vi "SerialWriteLines.vi"(8 "error in (no error)":errorcluster, 9 "REPL":string, 10 "Send":string, 11 "VISA Refnum in":refnum<visa-resource-name>) -> (0 "error out":errorcluster, 1 "Rest":string, 3 "VISA Refnum out":refnum<visa-resource-name>)   [LabVIEW 2020]
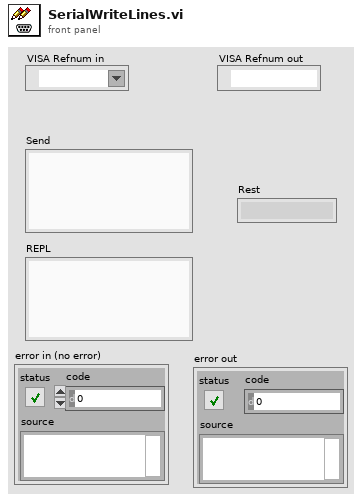
[diagram p1: front panel]
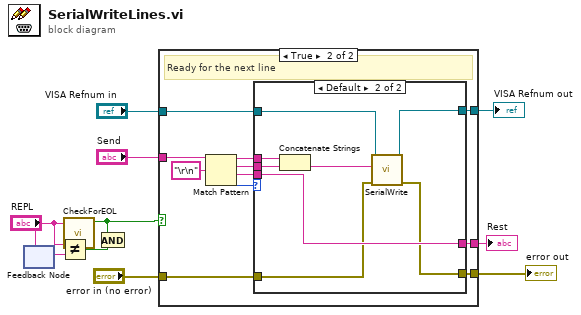
[diagram p0: block diagram]
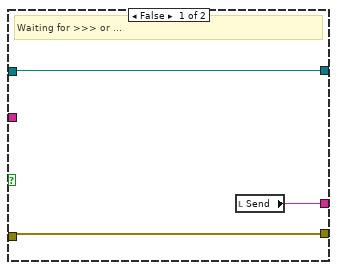
[diagram p2: hidden frame]
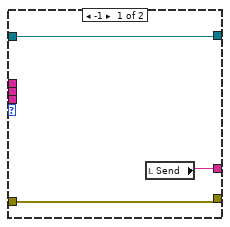
[diagram p3: hidden frame]
diagram:
  n1 = feedback-in #1("REPL") -> ()
  n2 = feedback #1() -> (w4:string)  [unwired: 1 in]
  n3 = Not Equal?(x="REPL", y=w4) -> (x != y?=w2:bool)
  n4 = call "CheckForEOL.vi"("REPL"="REPL") -> ("Complete?"=w1:bool)  [unwired: 10 in]
  n5 = And(x=w1, y=w2) -> ()  [unwired: 1 out]
  n6 = case shown="True" w1 {
    tunnel: "Send" -> [_ w23]
    tunnel: [w13 w19] -> w9
    tunnel: "VISA Refnum in" -> [w11 w17]
    tunnel: "error in (no error)" -> [w12 w16]
    tunnel: [w12 w15] -> w6
    tunnel: [w11 w14] -> w5
    frame False {
      # "Waiting for >>> or ..."
      n7 = local read "Send"() -> (w13:string)
    }
    frame True {
      # "Ready for the next line"
      n8 = Match Pattern(string=w23, regular expression="\r\n") -> (before substring=w24:string, match substring=w22:string, after substring=w18:string, offset past match=w20:i32)  [unwired: 1 in]
      n9 = case shown="Default" w20 {
        tunnel: w24 -> [_ w35]
        tunnel: w22 -> [_ w34]
        tunnel: w17 -> [w25 w32]
        tunnel: [w27 w33] -> w19
        tunnel: w18 -> [_ w33]
        tunnel: w16 -> [w26 w29]
        tunnel: [w26 w28] -> w15
        tunnel: [w25 w31] -> w14
        frame -1 {
          n10 = local read "Send"() -> (w27:string)
        }
        frame Default {
          n11 = Concatenate Strings(w35, w34) -> (w30:string)
          n12 = call "SerialWrite.vi"("error in (no error)"=w29, "Text"=w30, "VISA Refnum in"=w32) -> ("error out"=w28:errorcluster, "VISA Refnum out"=w31:refnum<visa-resource-name>)  [unwired: 7 in]
        }
      }
    }
  }
  "VISA Refnum out" <- w5
  "Rest" <- w9
  "error out" <- w6
